vi "Condition Poly VIs.vi"(8 "error in":errorcluster, 9 "Control FP Order":i32[](array[numeric]), 10 "Ref.Poly VIs":T1) -> (0 "error out":errorcluster)   [LabVIEW 2025, in "_Msg Rescript.lvlib" / "_Msg Rescript.lvclass"]
uses:
  _Msg Rescript.lvclass
  _Msg Rescript.lvclass/_Msg Rescript.ctl
  Poly VIs.ctl
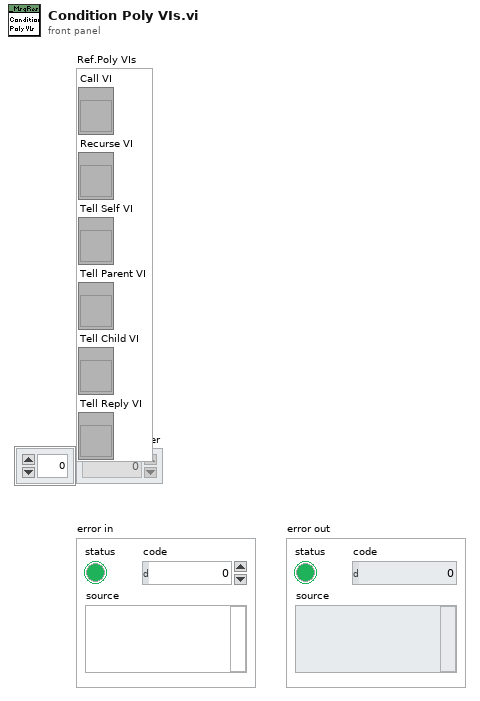
[diagram p1: front panel]
types:
  T1 = typedef "_Msg Rescript.lvlib/_Msg Rescript.lvclass/Poly VIs.ctl" = cluster{"Call VI":refnum<vi>, "Recurse VI":refnum<vi>, "Tell Self VI":refnum<vi>, "Tell Parent VI":refnum<vi>, "Tell Child VI":refnum<vi>, "Tell Reply VI":refnum<vi>}
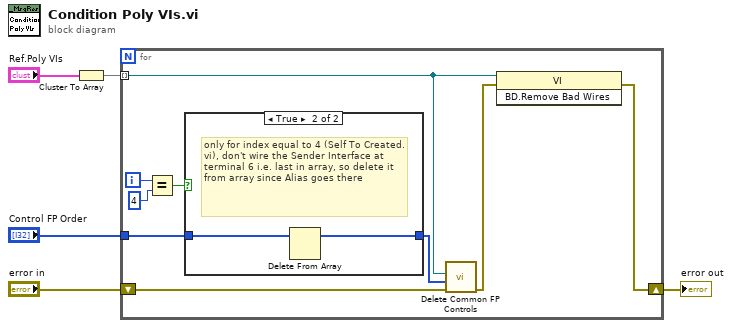
[diagram p0: block diagram]
diagram:
  n1 = Cluster To Array(cluster="Ref.Poly VIs") -> (array=w1:refnum<vi>[])
  n2 = for {
    tunnel: "Control FP Order" -> [w7]
    shift-right: [w12] -> w3
    shift-left: "error in" -> [w14]
    tunnel: w1 -> [w11] mode=indexing
    i -> [w8]
    n3 = Equal?(x=w8, y=4) -> (x = y?=w10:bool)
    n4 = case shown="True" w10 {
      tunnel: w7 -> [w15 w17]
      tunnel: [w15 w16] -> w6
      frame False {
      }
      frame True {
        # "only for index equal to 4 (Self To Created.vi), don't wire the Sender Interface at terminal 6 i.e. last in array, so delete it from array since Alias goes there"
        n5 = Delete From Array(array=w17) -> (array with subset deleted=w16:i32[])  [unwired: 2 in, 1 out]
      }
    }
    n6 = call "Delete Common FP Controls.vi"("error in"=w14, "Control FP Order"=w6, "Ref. VI"=w11) -> ("error out"=w13:errorcluster)  [unwired: 8 in]
    n7 = invoke class="VI" method="BD.Remove Bad Wires"(reference=w11, error in=w13) -> (error out=w12:errorcluster)  [unwired: 1 in, 2 out]
  }
  "error out" <- w3
